vi "MainVI.vi"() -> ()   [LabVIEW 2017]
uses:
  NameSurnameID.vi
panel:
  in  "Stop Main VI":bool
  in  "Tab Control":T1(tab)
  in  "Delete Measurement":bool
  out "Measurement data":string[][](table)
  in  "Select measurement:":u16(ring)
  out "Masurement Graph":waveform(dbl)(graph)
  in  "Refresh measurement list":bool
  in  "Display measurement":bool
  in  "Device name":string
  in  "Add device":bool
  out "Device list":string[][](array[string])
  in  "Select device:":u16(ring) items=["1: MyDaq", "2: MyRIO", "3: USB6001"]
  out "Current date and time":timestamp format="%<%H:%M\n%d/%m/%y>T"
  out "Waveform Chart":dbl(graph)
  in  "Save acquisition":bool
  in  "Stop acquisition":bool
  in  "Start acquisition":bool
  in  "Description":string
  in  "Measurement name":string
  out "Current user":string
  in  "Create new user":bool
  in  "Password":string
  in  "Username":string
  in  "Surname":string
  in  "Name":string
  in  "ChangePassword":bool
  in  "New password":string
  in  "Old password":string
  # "Add new device"
  # "Measurement information"
  # "Change password"
  # "Create new user"
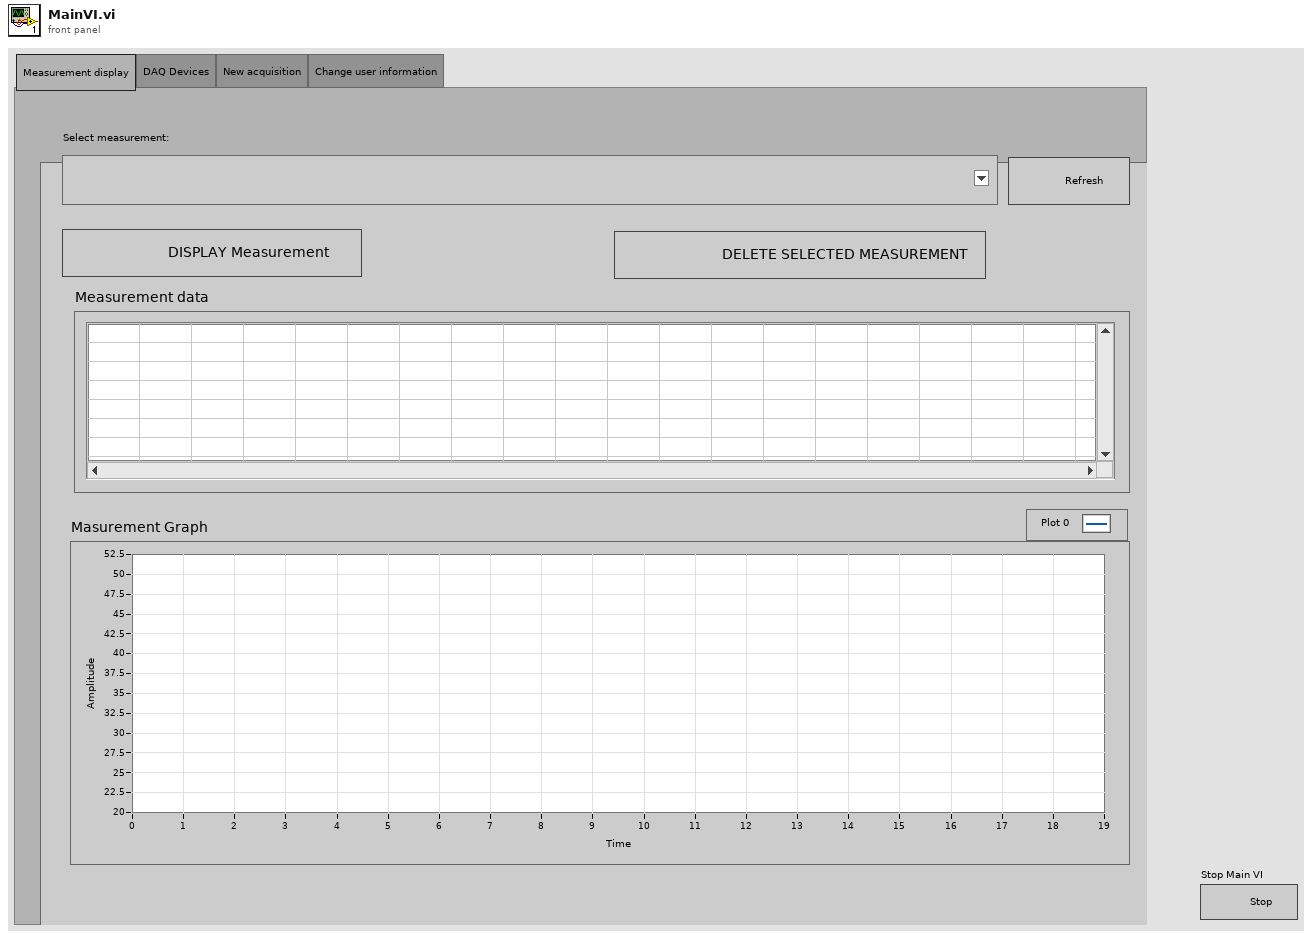
[diagram p1: front panel]
types:
  T1 = enum32{"Measurement display", "DAQ Devices", "New acquisition", "Change user information"}
  T2 = cluster{"userID":string, "password":string, "connection information":path}
  T3 = enum32{"Measurement display", "DAQ Devices", "Acquisition"}
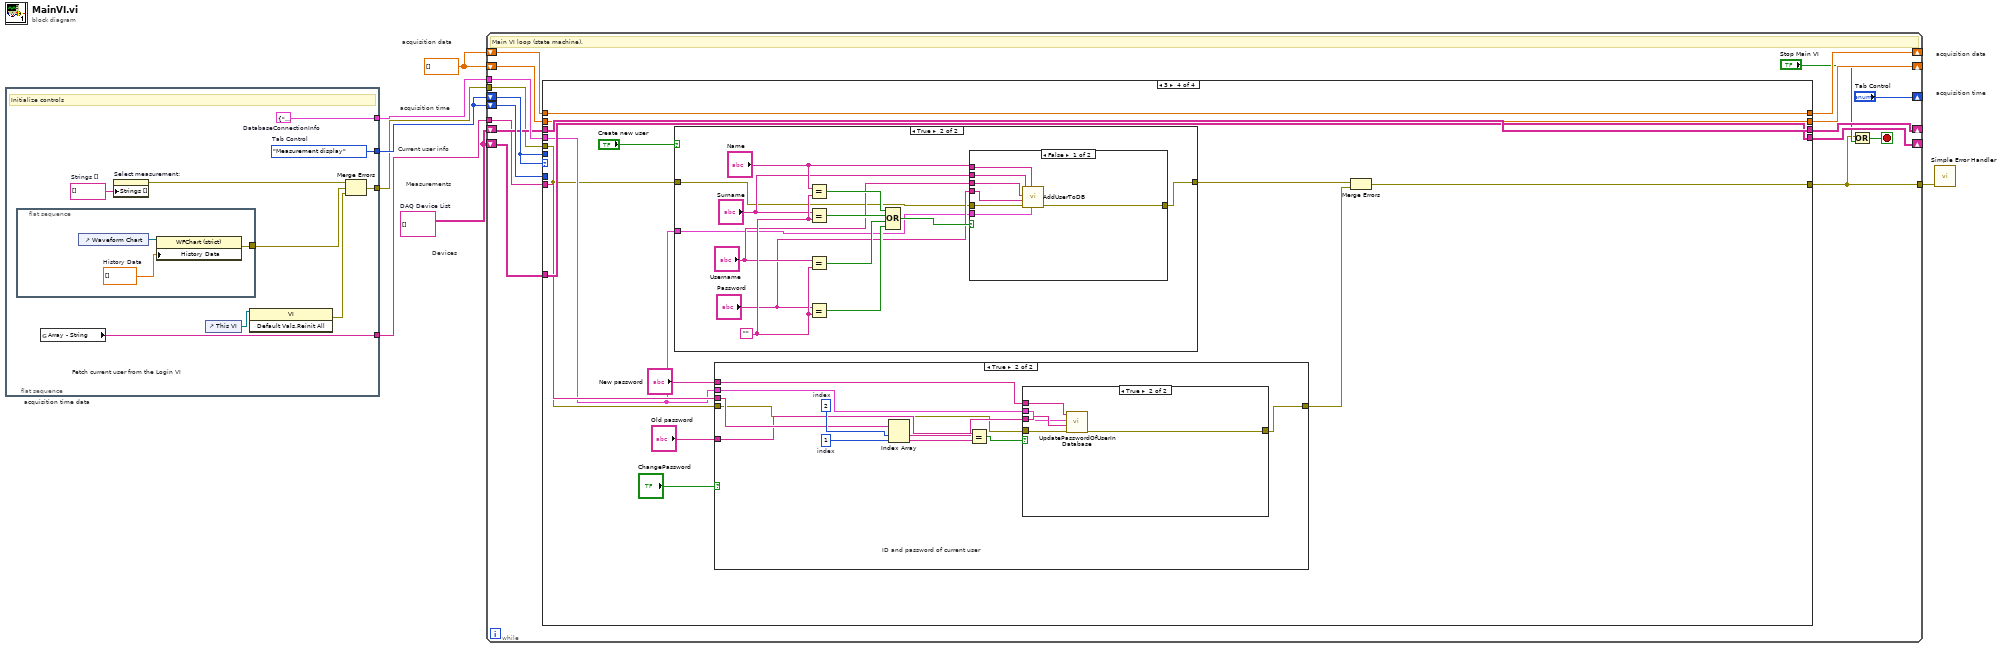
[diagram p0: block diagram]
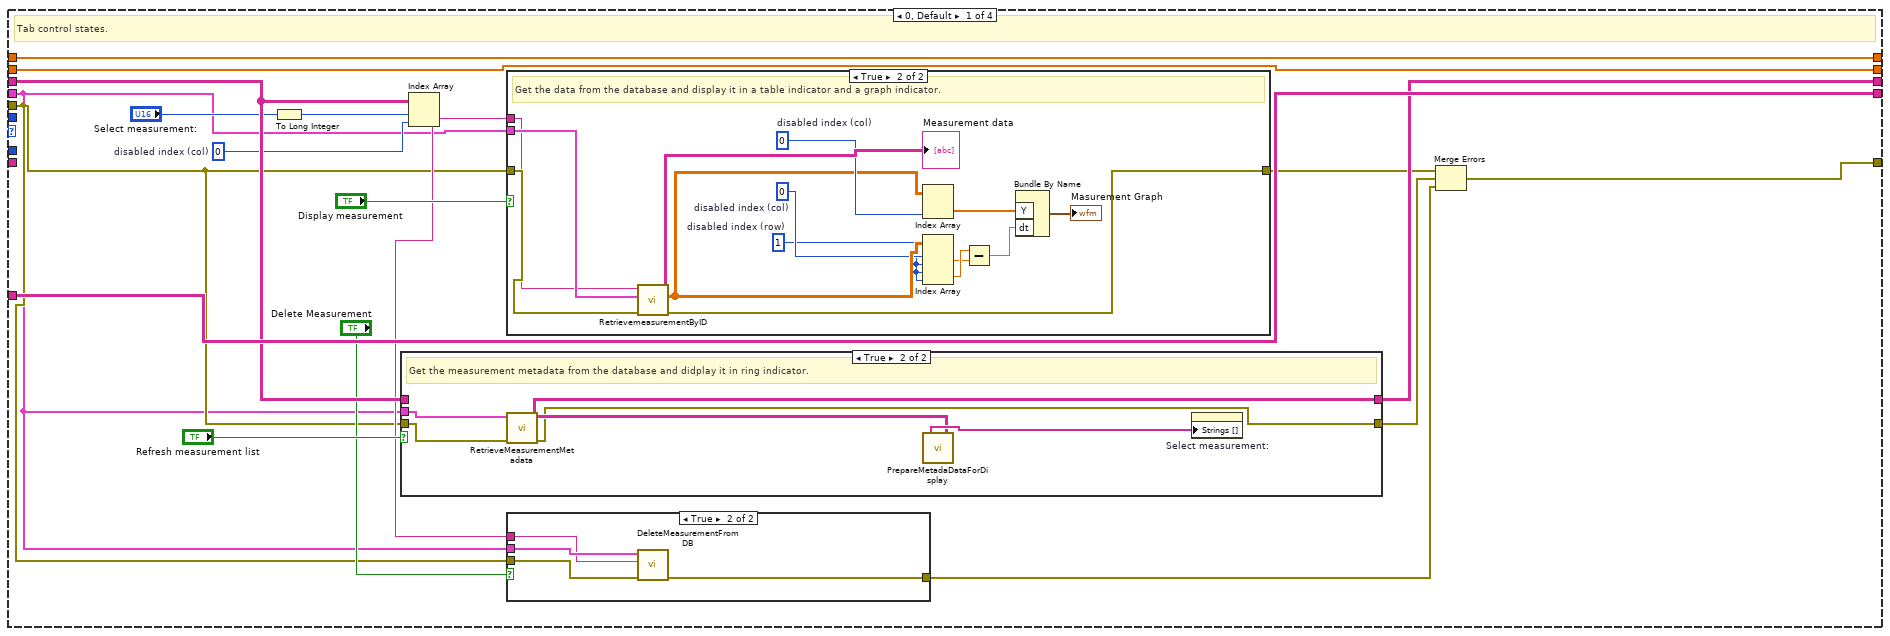
[diagram p2: hidden frame]
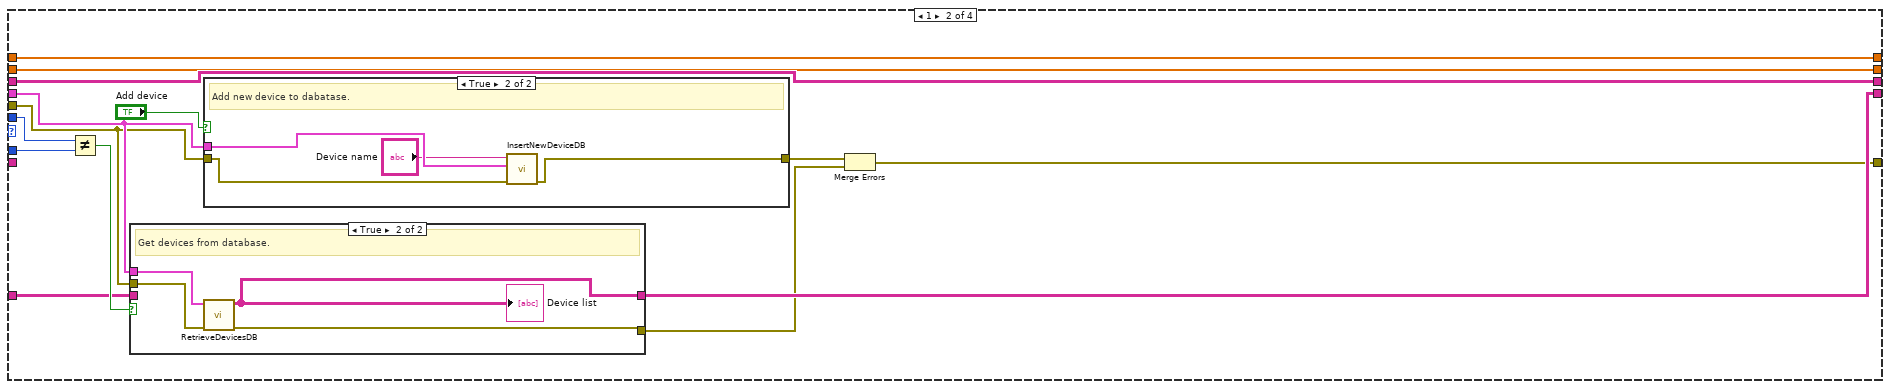
[diagram p6: hidden frame]
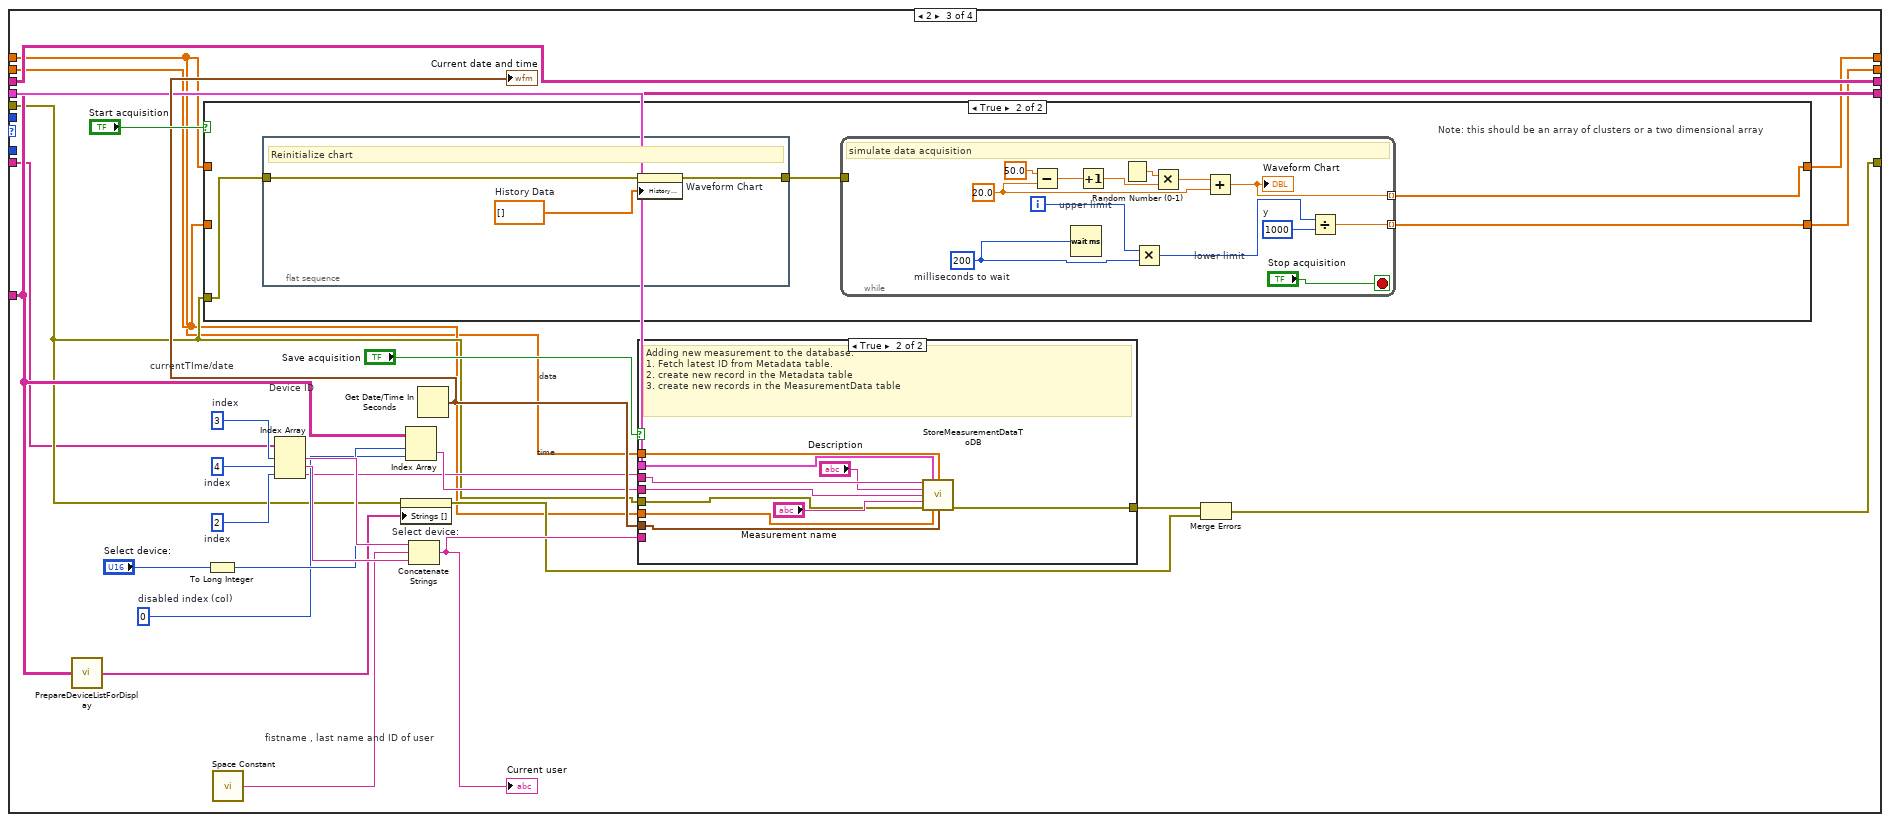
[diagram p9: hidden frame]
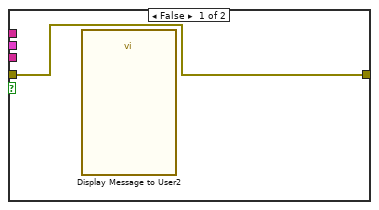
[diagram p13: hidden frame]
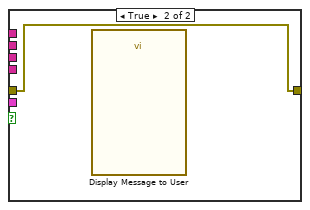
[diagram p15: hidden frame]
diagram:
  w2 = dbl[] []
  w5 = string[][] []  # DAQ Device List
  # "Current user info"
  # "acquisition data"
  # "acquisition time"
  # "acquisition time"
  # "acquisition time data"
  # "acquisition data"
  # "Devices"
  # "Measurements"
  n1 = flat-sequence {
    tunnel: [w16] -> w7
    tunnel: [w15] -> w6
    tunnel: [w9] -> w4
    tunnel: [w8] -> w1
    frame #0 {
      w13 = string[] []  # Strings []
      w15 = T2 {"userID"="Admin", "password"="", "connection information"=path "C:/Users/tnovak/Desktop/D.udl"}  # DatabaseConnectionInfo
      w16 = T3."Measurement display"  # Tab Control
      # "Fetch current user from the Login VI"
      # "Initialize controls"
      n2 = flat-sequence {
        tunnel: [w18] -> w11
        frame #0 {
          w19 = dbl[] []  # History Data
          n3 = control-ref of="Waveform Chart"() -> (w17:refnum<vi>)
          n4 = property on="Property Node" class="WFChart (strict)"(reference=w17, "History Data"=w19) -> (error out=w18:errorcluster)  [unwired: 1 in, 1 out]
        }
      }
      n5 = global read "NameSurnameID.vi" "Array - String"() -> (w8:string[])
      n6 = property on="Select measurement:" class="Ring (strict)"("Strings []"=w13) -> (error out=w12:errorcluster)  [unwired: 2 in, 1 out]
      n7 = control-ref of="This VI"() -> (w14:refnum<vi>)
      n8 = invoke class="VI" method="Default Vals.Reinit All"(reference=w14) -> (error out=w10:errorcluster)  [unwired: 2 in, 2 out]
      n9 = Merge Errors(w12, w11, w10) -> (w9:errorcluster)
    }
  }
  n10 = while {
    shift-right: ["Tab Control"] -> _
    shift-left: w7 -> [w31]
    shift-left: w7 -> [w36]
    tunnel: w6 -> [w35]
    shift-right: [w33] -> _
    shift-left: w5 -> [w34]
    shift-right: [w30] -> _
    shift-left: w5 -> [w29]
    shift-right: [w28] -> _
    shift-left: w2 -> [w26]
    shift-right: [w27] -> _
    shift-left: w2 -> [w25]
    tunnel: w4 -> [w24]
    tunnel: [w22] -> w3
    tunnel: w1 -> [w20]
    stop <- w21 stop-if-true
    # "Main VI loop (state machine)."
    n11 = case shown="3" w31 {
      tunnel: w31 -> [_ w94 _ _]
      tunnel: w36 -> [_ w93 _ _]
      tunnel: w35 -> [w37 w89 w124 w172]
      tunnel: w34 -> [w54 w91 w119 w179]
      tunnel: [w54 w90 w119 w179] -> w33
      tunnel: [w51 w88 w129 w180] -> w30
      tunnel: w29 -> [w50 w88 w129 w180]
      tunnel: [w48 w86 w115 w178] -> w28
      tunnel: [w49 w87 w114 w177] -> w27
      tunnel: w25 -> [w49 w87 w109 w177]
      tunnel: w26 -> [w48 w86 w108 w178]
      tunnel: w24 -> [w39 w85 w113 w171]
      tunnel: [w45 w82 w110 w168] -> w22
      tunnel: w20 -> [_ _ w107 w174]
      frame 0, Default {
        w41 = 0  # disabled index (col)
        # "Tab control states."
        n12 = To Long Integer(number="Select measurement:") -> (32bit integer=w43:i32)
        n13 = case shown="True" "Refresh measurement list" {
          tunnel: w37 -> [_ w81]
          tunnel: [w76 w79] -> w51
          tunnel: w50 -> [w76 _]
          tunnel: [w75 w78] -> w46
          tunnel: w39 -> [w75 w77]
          frame False {
          }
          frame True {
            # "Get the measurement metadata from the database and didplay it in ring indicator."
            n14 = call "RetrieveMeasurementMetadata.vi"("error in (no error)"=w77, "DatabaseConnectionInfo"=w81) -> ("error out"=w78:errorcluster, "MeasurementMetadata"=w79:string[][])  [unwired: 8 in]
            n15 = call "PrepareMetadaDataForDisplay.vi"("MeasurementMetadata"=w79) -> ("String array"=w80:string[])
            n16 = property on="Select measurement:" class="Ring (strict)"("Strings []"=w80) -> ()  [unwired: 2 in, 2 out]
          }
        }
        n17 = Index Array(array=w50, index (row)=w43, index (col)=w41) -> (element=w40:string)
        n18 = case shown="True" "Display measurement" {
          tunnel: w37 -> [_ w74]
          tunnel: w39 -> [w60 w63]
          tunnel: [w60 w62] -> w47
          tunnel: w40 -> [_ w61]
          frame False {
          }
          frame True {
            w68 = 1  # disabled index (row)
            w69 = 0  # disabled index (col)
            w72 = 0  # disabled index (col)
            # "Get the data from the database and display it in a table indicator and a graph indicator."
            n19 = call "RetrievemeasurementByID.vi"("error in (no error)"=w63, "DatabaseConnectionInfo"=w74, "ID"=w61) -> ("error out"=w62:errorcluster, "Double data"=w70:dbl[][], "String data"=→"Measurement data":string[][])  [unwired: 5 in, 1 out]
            n20 = Index Array(array=w70, index (col)=w72) -> (element=w71:dbl[])  [unwired: 1 in]
            n21 = Index Array(array=w70, index (row) #1=w69, index (col) #1=w68, index (row) #2=w68, index (col) #2=w68) -> (element #1=w66:dbl, element #2=w67:dbl)
            n22 = Subtract(x=w67, y=w66) -> (x-y=w65:dbl)
            n23 = Bundle By Name("Y"=w71, "dt"=w65) -> (→"Masurement Graph":waveform(dbl))  [unwired: 1 in]
          }
        }
        n24 = case shown="True" "Delete Measurement" {
          tunnel: w40 -> [_ w56]
          tunnel: [w55 w59] -> w38
          tunnel: w39 -> [w55 w57]
          tunnel: w37 -> [_ w58]
          frame False {
          }
          frame True {
            n25 = call "DeleteMeasurementFromDB.vi"("error in (no error)"=w57, "Measurement ID"=w56, "DatabaseConnectionInfo"=w58) -> ("error out"=w59:errorcluster)  [unwired: 8 in]
          }
        }
        n26 = Merge Errors(w47, w46, w38) -> (w45:errorcluster)
      }
      frame 1 {
        n27 = Not Equal?(x=w94, y=w93) -> (x != y?=w92:bool)
        n28 = case shown="True" w92 {
          tunnel: w89 -> [_ w101]
          tunnel: w91 -> [w97 _]
          tunnel: [w97 w100] -> w90
          tunnel: [w96 w99] -> w83
          tunnel: w85 -> [w96 w98]
          frame False {
          }
          frame True {
            # "Get devices from database."
            n29 = call "RetrieveDevicesDB.vi"("error in (no error)"=w98, "DatabaseConnectionInfo"=w101) -> ("error out"=w99:errorcluster, "Array"=w100:string[][])  [unwired: 8 in]
            "Device list" <- w100
          }
        }
        n30 = case shown="True" "Add device" {
          tunnel: w89 -> [_ w106]
          tunnel: [w102 w104] -> w84
          tunnel: w85 -> [w102 w103]
          frame False {
          }
          frame True {
            # "Add new device to dabatase."
            n31 = call "InsertNewDeviceDB.vi"("error in (no error)"=w103, "DatabaseConnectionInfo"=w106, "Device name"="Device name") -> ("error out"=w104:errorcluster)  [unwired: 8 in]
          }
        }
        n32 = Merge Errors(w84, w83) -> (w82:errorcluster)
      }
      frame 2 {
        w117 = 2  # index
        w120 = 0  # disabled index (col)
        w133 = 4  # index
        w134 = 3  # index
        # "time"
        # "data"
        # "currentTIme/date"
        # "Device ID"
        # "fistname , last name and ID of user"
        n33 = call "PrepareDeviceListForDisplay.vi"("DAQ Device List"=w119) -> ("PreparedDeviceListForDisplay"=w123:string[])
        n34 = case shown="True" "Start acquisition" {
          tunnel: [w147 w151] -> w115
          tunnel: [w146 w149] -> w114
          tunnel: w108 -> [w147 _]
          tunnel: w109 -> [w146 _]
          tunnel: w113 -> [_ w148]
          frame False {
          }
          frame True {
            # "Note: this should be an array of clusters or a two dimensional array"
            n35 = flat-sequence {
              tunnel: [w153] -> w150
              tunnel: w148 -> [w152]
              frame #0 {
                w154 = dbl[] []  # History Data
                # "Reinitialize chart"
                n36 = property on="Waveform Chart" class="WFChart (strict)"(error in=w152, "History Data"=w154) -> (error out=w153:errorcluster)  [unwired: 1 in, 1 out]
              }
            }
            n37 = while {
              tunnel: [w160] -> w151 mode=indexing
              tunnel: w150 -> [_]
              tunnel: [w155] -> w149 mode=indexing
              i -> [w159]
              stop <- "Stop acquisition" stop-if-true
              w156 = u32 1000  # y
              w161 = 20.0
              w158 = u32 200  # milliseconds to wait
              # "lower limit"
              # "upper limit"
              # "simulate data acquisition"
              n38 = Subtract(x=50.0, y=w161) -> (x-y=w164:dbl)
              n39 = Wait (ms)(milliseconds to wait=w158) -> ()  [unwired: 1 out]
              n40 = Increment(x=w164) -> (x+1=w163:dbl)
              n41 = Random Number (0-1)() -> (number: 0 to 1=w166:dbl)
              n42 = Multiply(x=w159, y=w158) -> (x*y=w157:u32)
              n43 = Multiply(x=w166, y=w163) -> (x*y=w162:dbl)
              n44 = Add(x=w162, y=w161) -> (x+y=w160:dbl)
              "Waveform Chart" <- w160
              n45 = Divide(x=w157, y=w156) -> (x/y=w155:dbl)
            }
          }
        }
        n46 = To Long Integer(number="Select device:") -> (32bit integer=w121:i32)
        n47 = call <vilib>:"Space Constant.vi"() -> ("String"=w130:string)
        n48 = Index Array(array=w107, index #1=w134, index #2=w133, index #3=w117) -> (element #1=w132:string, element #2=w131:string, element #3=w116:string)
        n49 = property on="Select device:" class="Ring (strict)"(error in=w113, "Strings []"=w123) -> (error out=w111:errorcluster)  [unwired: 1 in, 1 out]
        n50 = Index Array(array=w119, index (row)=w121, index (col)=w120) -> (element=w118:string)
        n51 = Concatenate Strings(w132, w130, w131) -> (w125:string)
        "Current user" <- w125
        n52 = Get Date/Time In Seconds() -> (seconds since 1Jan1904=w126:timestamp)
        "Current date and time" <- w126
        n53 = case shown="True" "Save acquisition" {
          tunnel: w126 -> [_ w144]
          tunnel: w125 -> [_ _]
          tunnel: w108 -> [_ w140]
          tunnel: w124 -> [_ w145]
          tunnel: w118 -> [_ w143]
          tunnel: w109 -> [_ w141]
          tunnel: w116 -> [_ w142]
          tunnel: w113 -> [w135 w137]
          tunnel: [w135 w136] -> w112
          frame False {
          }
          frame True {
            # "Adding new measurement to the database:\n1. Fetch latest ID from Metadata table.\n2. create new record in the Metadata table\n3. create new records in the MeasurementData table"
            n54 = call "StoreMeasurementDataToDB.vi"("UserID"=w142, "DatabaseConnectionInfo"=w145, "Data"=w140, "Description"="Description", "Device ID"=w143, "Measurement name"="Measurement name", "error in (no error)"=w137, "DataTimestamps"=w141, "seconds since 1Jan1904"=w144) -> ("error out"=w136:errorcluster)  [unwired: 6 in]
          }
        }
        n55 = Merge Errors(w112, w111) -> (w110:errorcluster)
      }
      frame 3 {
        n56 = case shown="True" "Create new user" {
          tunnel: w171 -> [w200 w203]
          tunnel: [w200 w202] -> w169
          tunnel: w172 -> [_ w201]
          frame False {
          }
          frame True {
            w213 = ""
            n57 = Equal?(x="Name", y=w213) -> (x = y?=w212:bool)
            n58 = Equal?(x="Surname", y=w213) -> (x = y?=w211:bool)
            n59 = Equal?(x="Username", y=w213) -> (x = y?=w210:bool)
            n60 = Equal?(x="Password", y=w213) -> (x = y?=w209:bool)
            n61 = Compound Arithmetic op=OR(w212, w211, w210, w209) -> (w208:bool)
            n62 = case shown="False" w208 {
              tunnel: "Name" -> [w219 _]
              tunnel: "Surname" -> [w218 _]
              tunnel: "Username" -> [w217 _]
              tunnel: "Password" -> [w216 _]
              tunnel: w203 -> [w220 w221]
              tunnel: [w215 w221] -> w202
              tunnel: w201 -> [w214 _]
              frame False {
                n63 = call "AddUserToDB.vi"("DatabaseConnectionInfo"=w214, "Name"=w219, "error in (no error)"=w220, "Password"=w216, "Username"=w217, "Surname"=w218) -> ("error out"=w215:errorcluster)  [unwired: 5 in]
              }
              frame True {
                n64 = call "Display Message to User"() -> ()  [unwired: 10 in, 2 out]
              }
            }
          }
        }
        n65 = case shown="True" "ChangePassword" {
          tunnel: "Old password" -> [_ w188]
          tunnel: w174 -> [_ w192]
          tunnel: "New password" -> [_ w187]
          tunnel: [w182 w185] -> w170
          tunnel: w172 -> [_ w184]
          tunnel: w171 -> [w182 w183]
          frame False {
          }
          frame True {
            w191 = 1  # index
            w193 = 2  # index
            # "ID and password of current user"
            n66 = Index Array(array=w192, index #1=w193, index #2=w191) -> (element #1=w186:string, element #2=w190:string)
            n67 = Equal?(x=w188, y=w190) -> (x = y?=w189:bool)
            n68 = case shown="True" w189 {
              tunnel: w187 -> [_ w198]
              tunnel: w186 -> [_ w199]
              tunnel: [w194 w197] -> w185
              tunnel: w184 -> [_ w196]
              tunnel: w183 -> [w194 w195]
              frame False {
                n69 = call "Display Message to User2"() -> ()  [unwired: 10 in, 2 out]
              }
              frame True {
                n70 = call "UpdatePasswordOfUserInDatabase.vi"("error in (no error)"=w195, "User ID"=w199, "DatabaseConnectionInfo"=w196, "New password"=w198) -> ("error out"=w197:errorcluster)  [unwired: 7 in]
              }
            }
          }
        }
        n71 = Merge Errors(w169, w170) -> (w168:errorcluster)
      }
    }
    n72 = Or(x=w22, y="Stop Main VI") -> (x .or. y?=w21:bool)
  }
  n73 = call <vilib>:"Simple Error Handler.vi"("error in (no error)"=w3) -> ()  [unwired: 4 in, 5 out]
